vi "Create Canonicalized Headers.vi"(10 "HTTP Session in":refnum<class "Session.lvclass">) -> (2 "Canonical headers":string, 3 "HTTP Session out":refnum<class "Session.lvclass">)   [LabVIEW 2015, in "NI_Azure_Core.lvlib" / "Session.lvclass"]
uses:
  Session.lvclass
  Name Value Pair.ctl
  Session.lvclass/Session.ctl
  Read HTTP Session.vi
  Read Request Headers.vi
  <vilib>/httpClient/LabVIEWHTTPClient.lvlib
  NI_Azure_Core.lvlib
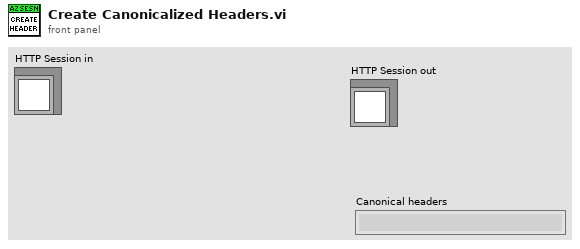
[diagram p1: front panel]
types:
  T1 = typedef "NI_Azure_Core.lvlib/Name Value Pair.ctl" = cluster{"name":string, "value":string}
  T2 = typedef "LVDateTimeRec.ctl" = cluster{"fractional second":dbl, "second":i32, "minute":i32, "hour":i32, "day of month":i32, "month":i32, "year":i32, "day of week":i32, "day of year":i32, "DST":i32}
  T3 = typedef "LabVIEWHTTPClient.lvlib/ClientHandle.ctl" = refnum<k1>
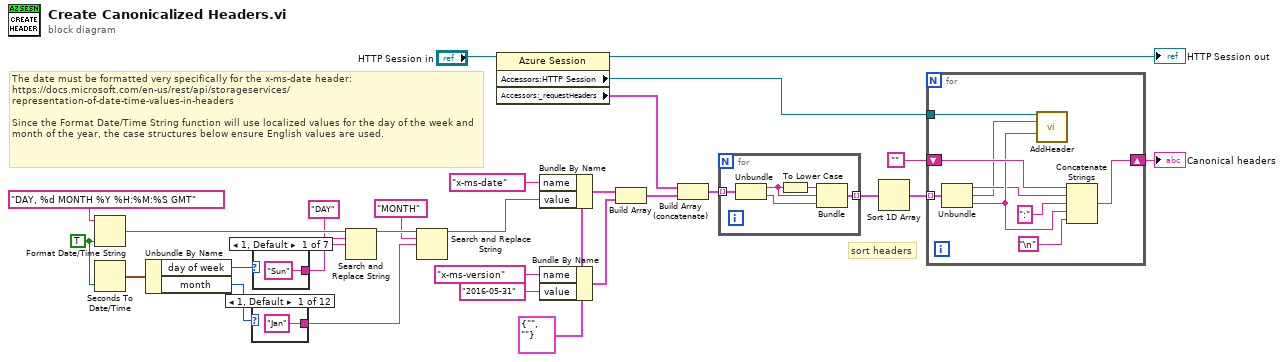
[diagram p0: block diagram]
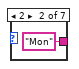
[diagram p2: hidden frame]
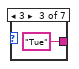
[diagram p3: hidden frame]
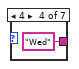
[diagram p4: hidden frame]
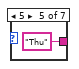
[diagram p5: hidden frame]
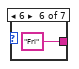
[diagram p6: hidden frame]
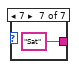
[diagram p7: hidden frame]
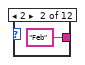
[diagram p8: hidden frame]
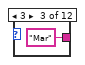
[diagram p9: hidden frame]
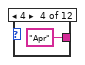
[diagram p10: hidden frame]
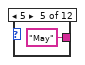
[diagram p11: hidden frame]
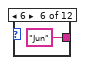
[diagram p12: hidden frame]
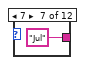
[diagram p13: hidden frame]
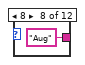
[diagram p14: hidden frame]
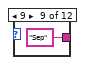
[diagram p15: hidden frame]
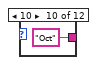
[diagram p16: hidden frame]
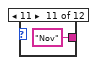
[diagram p17: hidden frame]
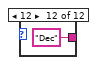
[diagram p18: hidden frame]
diagram:
  w11 = TRUE ("UTC format")
  w14 = T1 {"name"="", "value"=""} ("Name Value Pair")
  # "The date must be formatted very specifically for the x-ms-date header:\nhttps://docs.microsoft.com/en-us/rest/api/storageservices/representation-of-date-time-values-in-headers\n\nSince the Format Date/Time String function will use localized values for the day of the week and month of the year, the case structures below ensure English values are used."
  # "sort headers"
  n1 = Format Date/Time String(time format string (%c)="DAY, %d MONTH %Y %H:%M:%S GMT", UTC format=w11) -> (date/time string=w9:string)  [unwired: 1 in]
  n2 = Seconds To Date/Time(to UTC (F)=w11) -> (date time rec=w10:T2)  [unwired: 1 in]
  n3 = Unbundle By Name(w10) -> ("day of week"=w5:i32, "month"=w3:i32)
  n4 = case shown="1, Default" w3 {
    tunnel: ["Jan" "Feb" "Mar" "Apr" "May" "Jun" "Jul" "Aug" "Sep" "Oct" "Nov" "Dec"] -> w2
    frame 1, Default {
    }
    frame 2 {
    }
    frame 3 {
    }
    frame 4 {
    }
    frame 5 {
    }
    frame 6 {
    }
    frame 7 {
    }
    frame 8 {
    }
    frame 9 {
    }
    frame 10 {
    }
    frame 11 {
    }
    frame 12 {
    }
  }
  n5 = case shown="1, Default" w5 {
    tunnel: ["Sun" "Mon" "Tue" "Wed" "Thu" "Fri" "Sat"] -> w4
    frame 1, Default {
    }
    frame 2 {
    }
    frame 3 {
    }
    frame 4 {
    }
    frame 5 {
    }
    frame 6 {
    }
    frame 7 {
    }
  }
  n6 = Search and Replace String(input string=w9, search string="DAY", replace string=w4) -> (result string=w7:string)  [unwired: 5 in, 3 out]
  n7 = Search and Replace String(input string=w7, search string="MONTH", replace string=w2) -> (result string=w1:string)  [unwired: 5 in, 3 out]
  n8 = property class="Azure Session"(reference="HTTP Session in") -> (reference out=→"HTTP Session out":refnum<class "Session.lvclass">, "Accessors:HTTP Session"=w22:T3, "Accessors:_requestHeaders"=w13:T1[])  [unwired: 1 in, 1 out]
  n9 = Bundle By Name(cluster=w14, "name"="x-ms-date" ("header"), "value"=w1) -> (w18:T1)
  n10 = Bundle By Name(cluster=w14, "name"="x-ms-version" ("header"), "value"="2016-05-31") -> (w15:T1)
  n11 = Build Array(w18, w15) -> (w20:T1[])
  n12 = Build Array (concatenate)(w13, w20) -> (w25:T1[])
  n13 = for {
    tunnel: w25 -> [w52] mode=indexing
    tunnel: [w49] -> w24 mode=indexing
    n14 = Unbundle(w52) -> ("name"=w50:string, "value"=w48:string)
    n15 = To Lower Case(string=w50) -> (all lower case string=w51:string)
    n16 = Bundle(w51, "name"=w50, "value"=w48) -> (w49:cluster{string, "name":string, "value":string})  [unwired: 1 in]
  }
  n17 = Sort 1D Array(array=w24) -> (sorted array=w28:cluster{string, "name":string, "value":string}[])
  n18 = for {
    tunnel: w28 -> [w61] mode=indexing
    shift-right: [w57] -> w26
    shift-left: "" -> [w58]
    tunnel: w22 -> [w56]
    n19 = Unbundle(w61) -> (w54:string, "name"=w53:string, "value"=w55:string)
    n20 = call <vilib>:"AddHeader.vi"("client handle"=w56, "header"=w53, "value"=w55) -> ()  [unwired: 11 in, 2 out]
    n21 = Concatenate Strings(w58, w54, ":", w55, "\n") -> (w57:string)
  }
  "Canonical headers" <- w26
